vi "Trivariate Joint Normal Distribution_PN.vi"(7 "invSqrtpix23":dbl, 8 "W":dbl, 9 "V":dbl, 10 "U":dbl, 11 "Current stats":dbl[](array[numeric])=[0.0, 0.0, 0.0, 0.0, 0.0, 0.0, 0.0, 0.0]) -> (3 "F(U, V, W)":dbl)   [LabVIEW 2010]
panel:
  # "U\nV\nW\nu^2\nv^2\nw^2\nuv\nuw\nvw"
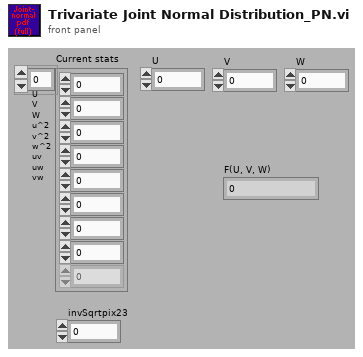
[diagram p1: front panel]
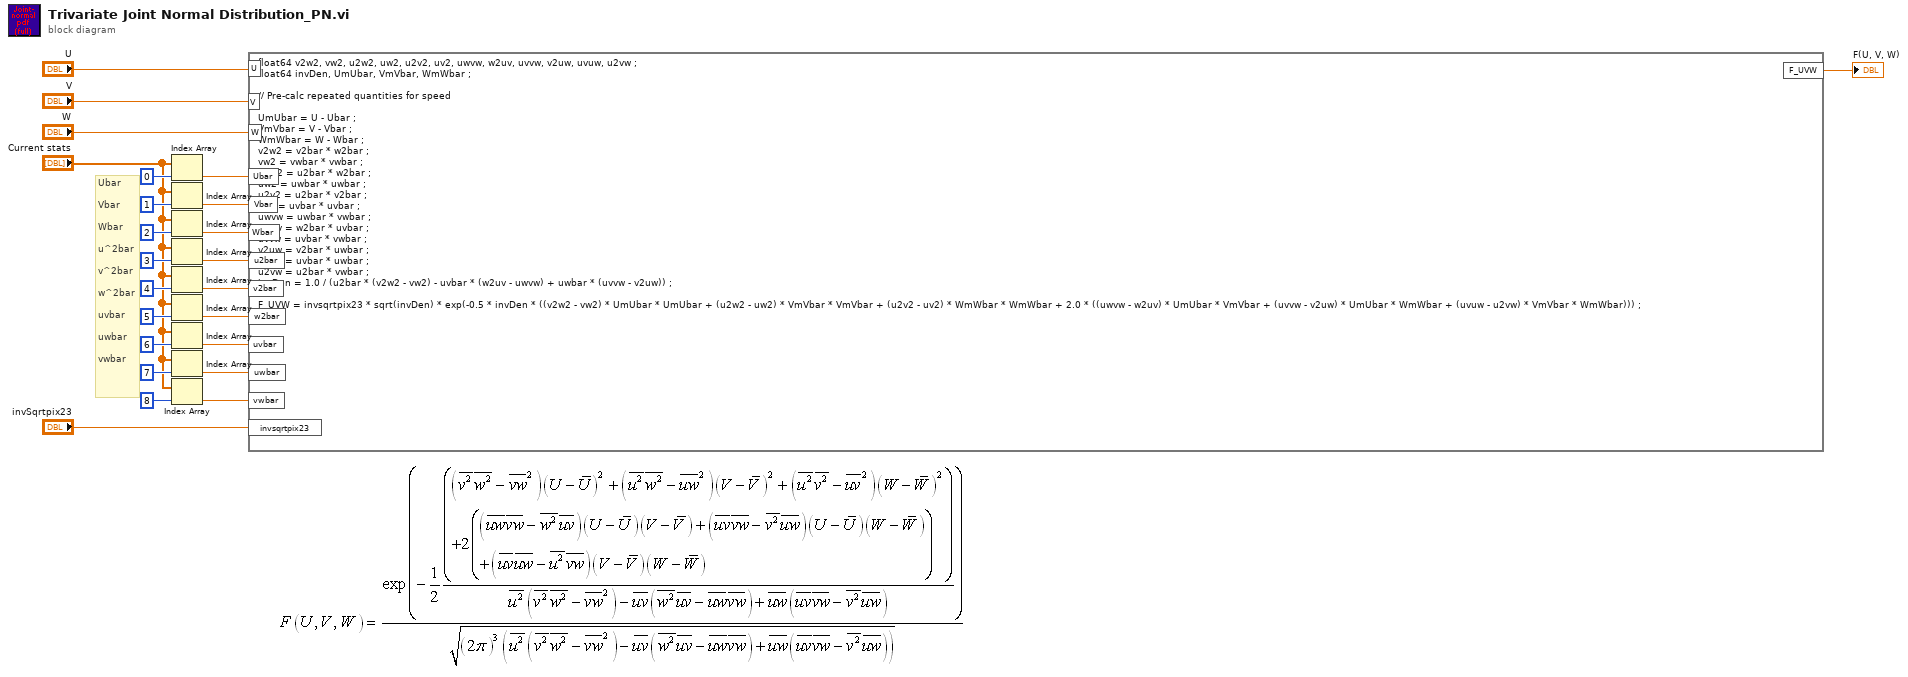
[diagram p0: block diagram]
diagram:
  # "Ubar\n\nVbar\n\nWbar\n\nu^2bar\n\nv^2bar\n\nw^2bar\n\nuvbar\n\nuwbar\n\nvwbar"
  n1 = Index Array(array="Current stats", index=0) -> (element=w16:dbl)
  n2 = Index Array(array="Current stats", index=1) -> (element=w15:dbl)
  n3 = Index Array(array="Current stats", index=2) -> (element=w2:dbl)
  n4 = Index Array(array="Current stats", index=3) -> (element=w3:dbl)
  n5 = Index Array(array="Current stats", index=4) -> (element=w4:dbl)
  n6 = Index Array(array="Current stats", index=5) -> (element=w5:dbl)
  n7 = Index Array(array="Current stats", index=6) -> (element=w6:dbl)
  n8 = Index Array(array="Current stats", index=7) -> (element=w7:dbl)
  n9 = Index Array(array="Current stats", index=8) -> (element=w9:dbl)
  n10 = formula code="float64 v2w2, vw2, u2w2, uw2, u2v2, uv2, uwvw, w2uv, uvvw, v2uw, uvuw, u2vw ;\nfloat64 invDen, UmUbar, VmVbar, WmWbar ;\n\n// Pre-calc repeated quantities for speed\n\nUmUbar = U - Ubar ;\nVmVbar = V - Vbar ;\nWmWbar = W - Wbar ;\nv2w2 = v2bar * w2bar ;\nvw2 = vwbar * vwbar ;\nu2w2 = u2bar * w2bar ;\nuw2 = uwbar * uwbar ;\nu2v2 = u2bar * v2bar ;\nuv2 = uvbar * uvbar ;\nuwvw = uwbar * vwbar ;\nw2uv = w2bar * uvbar ;\nuvvw = uvbar * vwbar ;\nv2uw = v2bar * uwbar ;\nuvuw = uvbar * uwbar ;\nu2vw = u2bar * vwbar ;\ninvDen = 1.0 / (u2bar * (v2w2 - vw2) - uvbar * (w2uv - uwvw) + uwbar * (uvvw - v2uw)) ;\n\nF_UVW = invsqrtpix23 * sqrt(invDen) * exp(-0.5 * invDen * ((v2w2 - vw2) * UmUbar * UmUbar + (u2w2 - uw2) * VmVbar * VmVbar + (u2v2 - uv2) * WmWbar * WmWbar + 2.0 * ((uwvw - w2uv) * UmUbar * VmVbar + (uvvw - v2uw) * UmUbar * WmWbar + (uvuw - u2vw) * VmVbar * WmWbar))) ;"("Ubar"=w16, "Vbar"=w15, "u2bar"=w3, "v2bar"=w4, "w2bar"=w5, "uvbar"=w6, "uwbar"=w7, "vwbar"=w9, "U"="U", "V"="V", "W"="W", "Wbar"=w2, "invsqrtpix23"="invSqrtpix23") -> ("F_UVW"=→"F(U, V, W)":dbl)
